vi "Simulator1.vi"() -> ()   [LabVIEW 2014]
panel:
  out "Output":dbl format="%#_13g"
  out "path":path
  in  "Input":dbl format="%#_13g"
  in  "Action":string
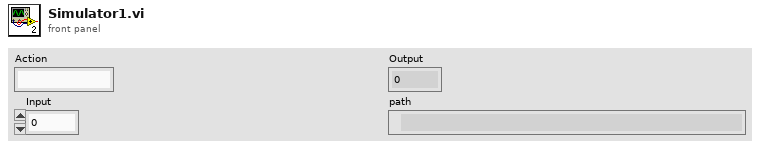
[diagram p1: front panel]
types:
  T1 = enum16{"open", "replace", "create", "open or create", "replace or create", "replace or create with confirmation"}
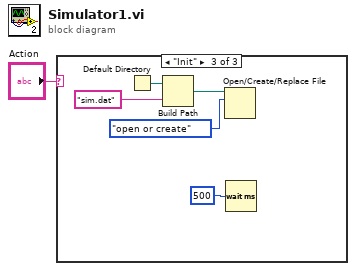
[diagram p0: block diagram]
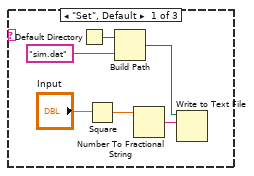
[diagram p2: hidden frame]
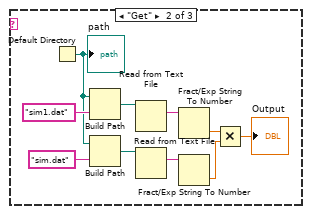
[diagram p3: hidden frame]
diagram:
  n1 = case shown="\"Init\"" "Action" {
    frame "Set", Default {
      n2 = Default Directory() -> (w4:path)
      n3 = Square(x="Input") -> (x^2=w3:dbl)
      n4 = Build Path(base path=w4, name or relative path="sim.dat") -> (appended path=w6:path)
      n5 = Number To Fractional String(number=w3) -> (F-format string=w5:string)  [unwired: 3 in]
      n6 = Write to Text File(file (use dialog)=w6, text=w5) -> ()  [unwired: 2 in, 3 out]
    }
    frame "Get" {
      n7 = Default Directory() -> (w9:path)
      "path" <- w9
      n8 = Build Path(base path=w9, name or relative path="sim1.dat") -> (appended path=w11:path)
      n9 = Build Path(base path=w9, name or relative path="sim.dat") -> (appended path=w16:path)
      n10 = Read from Text File(file (use dialog)=w11) -> (text=w10:string)  [unwired: 3 in, 3 out]
      n11 = Read from Text File(file (use dialog)=w16) -> (text=w15:string)  [unwired: 3 in, 3 out]
      n12 = Fract/Exp String To Number(string=w10) -> (number=w8:dbl)  [unwired: 3 in, 1 out]
      n13 = Fract/Exp String To Number(string=w15) -> (number=w14:dbl)  [unwired: 3 in, 1 out]
      n14 = Multiply(x=w8, y=w14) -> (x*y=→"Output":dbl)
    }
    frame "Init" {
      n15 = Default Directory() -> (w19:path)
      n16 = Build Path(base path=w19, name or relative path="sim.dat") -> (appended path=w21:path)
      n17 = Open/Create/Replace File(file path (use dialog)=w21, operation (0:open)=T1."open or create") -> ()  [unwired: 4 in, 3 out]
      n18 = Wait (ms)(milliseconds to wait=u32 500) -> ()  [unwired: 1 out]
    }
  }
